vi "getTelElement.vi"(8 "error in (no error)":errorcluster, 10 "queueTcpClientFromDdsTimeout":i32, 11 "TcpServer in":refnum<class "TcpServer.lvclass">) -> (0 "error out":errorcluster, 1 "Remaining Elements":i32, 2 "tcpPacket":string, 3 "TcpServer out":refnum<class "TcpServer.lvclass">)   [LabVIEW 2018, in "TcpServer.lvclass"]
doc: "Get telemetry elements one by one from queueTcpClientFromDds. Timeout is set in configServer.vi but you can modify this timeout through the queueTcpClientFromDdsTimeout control.\n\nNote: this function will not handle any error internally, so the user must handle the errors when call it."
uses:
  TcpServer.lvclass
  TcpServer.lvclass/TcpServer.ctl
  TcpServerTel/TcpServerTel.lvclass
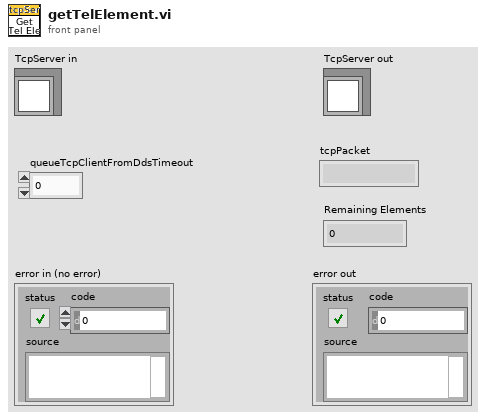
[diagram p1: front panel]
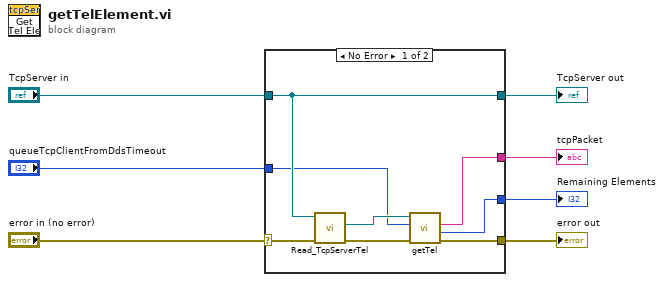
[diagram p0: block diagram]
diagram:
  n1 = case shown="No Error" "error in (no error)" {
    selector: "error in (no error)" -> [w15 w16]
    tunnel: [w11 w16] -> w7
    tunnel: "TcpServer in" -> [w14 w17]
    tunnel: [w14 w17] -> w4
    tunnel: "queueTcpClientFromDdsTimeout" -> [w10 _]
    tunnel: [w9 _] -> w2
    tunnel: [w8 _] -> w1
    frame No Error {
      n2 = call "Read_TcpServerTel.vi"("error in (no error)"=w15, "TcpServer in"=w14) -> ("error out"=w12:errorcluster, "TcpServerTel.lvclass"=w13:refnum<class "TcpServerTel.lvclass">)  [unwired: 7 in, 1 out]
      n3 = call "getTel.vi"("error in (no error)"=w12, "queueTcpClientFromDdsTimeout"=w10, "tcpServerTel in"=w13) -> ("error out"=w11:errorcluster, "Remaining Elements"=w8:i32, "tcpPacket"=w9:string)  [unwired: 5 in, 1 out]
    }
    frame Error {
    }
  }
  "error out" <- w7
  "TcpServer out" <- w4
  "tcpPacket" <- w2
  "Remaining Elements" <- w1
